vi "SignalAnalysisFrames.vi"() -> ()   [LabVIEW 2019]
uses:
  <vilib>/Analysis/4window.llb/windowTd.ctl
  <vilib>/Analysis/baseanly.llb/Mean (DBL).vi
  <vilib>/measure/maspectr.llb/FFT Spectrum (Mag-Phase) for N Chan.vi
  <vilib>/addons/Sound and Vibration/Order Analysis/Tach Process/OAT Analog Tacho Process (1 Tacho).vi
  <vilib>/addons/Sound and Vibration/Order Analysis/Resample Order Tracking/OAT Convert to Even Angle Signal (N Channels).vi
  <vilib>/addons/Sound and Vibration/Order Analysis/Utility/OAT Output Triggered Even Angle Signal (N Channels).vi
  <vilib>/addons/Sound and Vibration/Order Analysis/Resample Order Tracking/OAT Order Power Spectrum (N Channels).vi
  <vilib>/Analysis/NI_AALPro.lvlib
  <vilib>/measure/NI_MAPro.lvlib
  <vilib>/Analysis/NI_AALBase.lvlib
  <vilib>/addons/Sound and Vibration/Order Analysis/Tach Process/SoundVib_TachProcess.lvlib
  <vilib>/addons/Sound and Vibration/Order Analysis/Resample Order Tracking/SoundVib_OrderTracking.lvlib
  <vilib>/addons/Sound and Vibration/Order Analysis/Utility/SoundVib_OAUtility.lvlib
panel:
  out "Rotational speed [RPM] 2":dbl format="%0.2f"
  out "Rotational speed [RPM]":dbl format="%0.2f"
  in  "dł. ramki [s]":dbl=1.0
  in  "czułość 2 [V/g]":dbl=0.206
  in  "Skalować sygnał 2?":bool=TRUE
  in  "file path 2":path
  out "FFT analizator":cluster{"f0":dbl, "df":dbl, "magnitude":dbl[]}[](graph)
  out "order power spectrum 2":T1(graph)
  in  "FFT averaging":T2={"averaging mode"=enum."Vector averaging", "weighting mode"=enum."Exponential", "number of averages"=10}
  in  "Skalować sygnał 1?":bool
  out "order power spectrum":T1(graph)
  out "FFT karta pomiarowa":cluster{"f0":dbl, "df":dbl, "magnitude":dbl[]}[](graph)
  in  "order resolution":dbl=0.1 min=0.0 format="%.2f"
  in  "pulse/revolution (1)":i32=4
  in  "czułość 1 [V/g]":dbl=1.0
  in  "fs [Hz]":i64=5120
  in  "file path":path
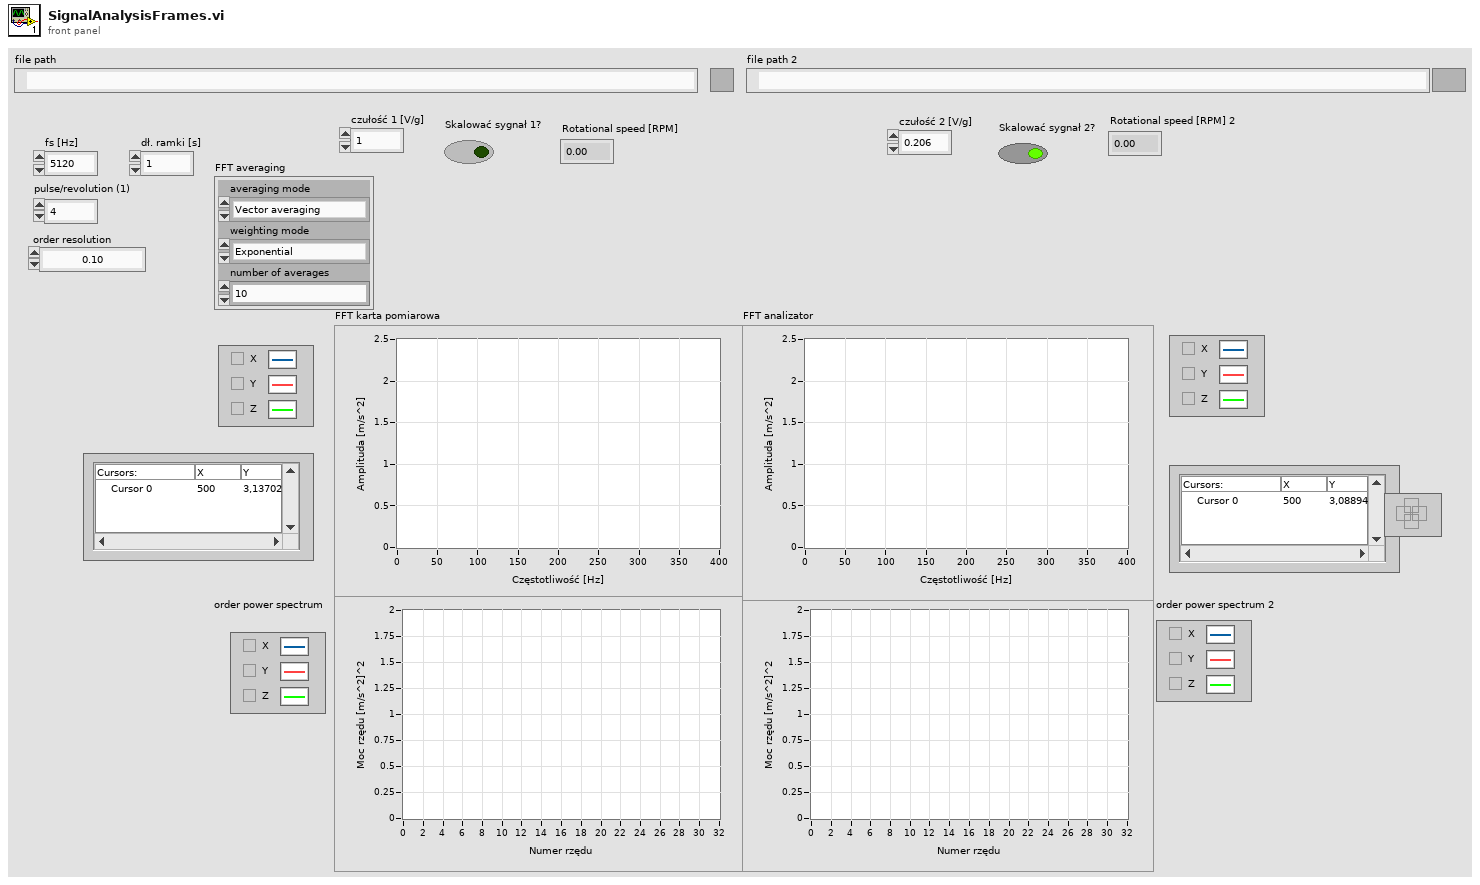
[diagram p1: front panel]
types:
  T1 = cluster{"order 0":dbl, "delta order":dbl, "magnitude":dbl[]}[]
  T2 = cluster{"averaging mode":enum16{"No averaging", "Vector averaging", "RMS averaging", "Peak hold"}, "weighting mode":enum16{"Linear", "Exponential"}, "number of averages":u32}
  T3 = enum16{"open", "open or create", "create or replace", "create", "open (read-only)"}
  T4 = enum16{"No averaging", "Vector averaging", "RMS averaging", "Peak hold"}
  T5 = cluster{"averaging mode":enum16{"No averaging", "Vector averaging", "RMS averaging", "Peak hold"}, "weighting mode":enum16{"Linear", "Exponential"}, "number of averages":u32, "linear mode":enum16{"One shot", "Auto restart"}}
  T6 = typedef "NI_AALPro.lvlib/windowTd.ctl" = u32
  T7 = typedef "SoundVib_TachProcess.lvlib/speed profile.ctl" = cluster{"time [s]":dbl[], "speed [RPM]":dbl[]}
  T8 = typedef "svc_Resampled Channel Info.ctl" = cluster{"channel name":string, "description":string, " channel info":T9}
  T9 = typedef "svc_Channel Info.ctl" = cluster{"sensor sensitivity":dbl, "engineering units":T10, "dB reference":dbl, "custom label":string, "weighting filter":T11, "pregain":dbl}
  T10 = typedef "svc_Engineering Units Text Ring.ctl" = u16
  T11 = typedef "svc_Weighting Filter Text Ring.ctl" = u16
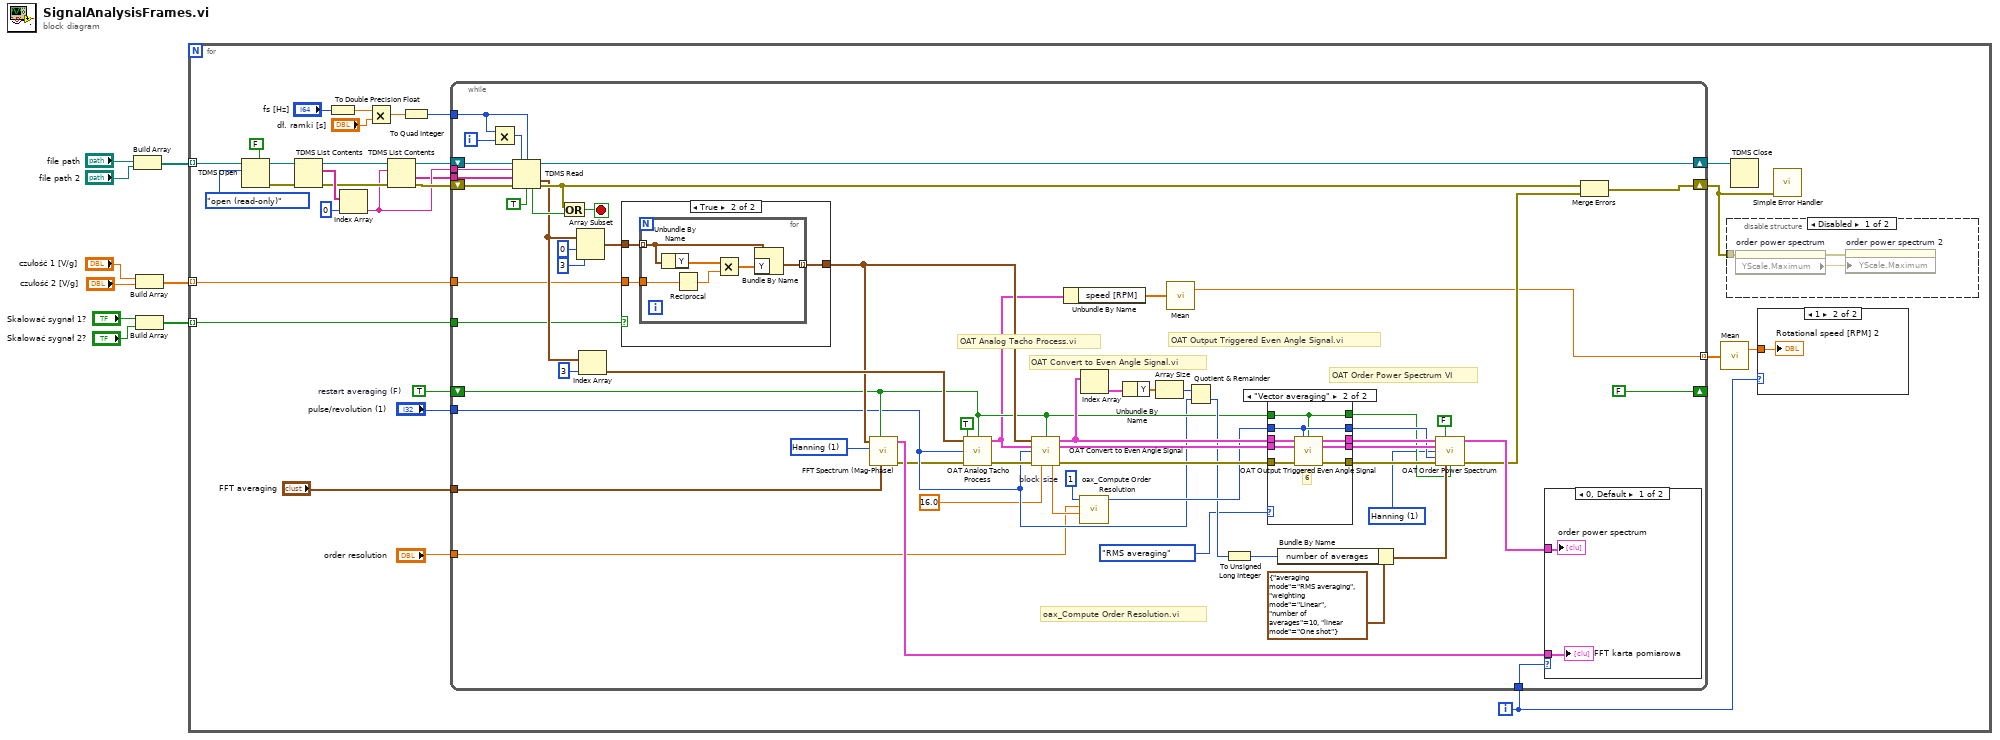
[diagram p0: block diagram]
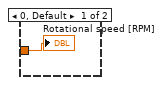
[diagram p3: hidden frame]
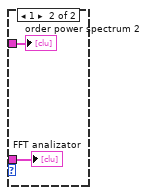
[diagram p5: hidden frame]
diagram:
  n1 = Build Array("file path", "file path 2") -> (w5:path[])
  n2 = Build Array("czułość 1 [V/g]", "czułość 2 [V/g]") -> (w3:dbl[])
  n3 = Build Array("Skalować sygnał 1?", "Skalować sygnał 2?") -> (w1:bool[])
  n4 = for {
    tunnel: w3 -> [w23] mode=indexing
    tunnel: w1 -> [w20] mode=indexing
    tunnel: w5 -> [w19] mode=indexing
    i -> [w12]
    w24 = TRUE  # restart averaging (F)
    n5 = TDMS Open(5:FALSE ("create index file? (T)"), 10:T3."open (read-only)" ("operation (0:open)"), 11:w19) -> (0:w28:errorcluster, 3:w29:refnum<k34>)  [unwired: 4 in]
    n6 = TDMS List Contents(4:w28, 7:w29) -> (0:w33:errorcluster, 2:w36:string[], 3:w35:refnum<k34>)  [unwired: 1 in, 1 out]
    n7 = To Double Precision Float(number="fs [Hz]") -> (double precision float=w15:dbl)
    n8 = Index Array(array=w36, index=0) -> (element=w31:string)
    n9 = Multiply(x=w15, y="dł. ramki [s]") -> (x*y=w18:dbl)
    n10 = TDMS List Contents(4:w33, 6:w31, 7:w35) -> (0:w32:errorcluster, 1:w30:string[], 3:w34:refnum<k34>)  [unwired: 1 out]
    n11 = To Quad Integer(1:w18) -> (0:w16:i64)
    n12 = while {
      tunnel: w31 -> [w101]
      tunnel: w30 -> [w100]
      shift-right: [w98] -> w27
      shift-left: w34 -> [w103]
      shift-right: [w83] -> w11
      shift-left: w32 -> [w102]
      tunnel: w16 -> [w92]
      shift-right: [FALSE ("restart averaging (F)")] -> _
      shift-left: w24 -> [w55]
      tunnel: w23 -> [w84]
      tunnel: "pulse/revolution (1)" -> [w54]
      tunnel: "order resolution" -> [w51]
      tunnel: w20 -> [w82]
      tunnel: "FFT averaging" -> [w81]
      tunnel: w12 -> [w79]
      tunnel: [w44] -> w14 mode=indexing
      i -> [w94]
      stop <- w97 stop-if-true
      w49 = u32 1 items=["None"=0, "Hanning"=1, "Hamming"=2, "Blackman-Harris"=3, "Exact Blackman"=4, "Blackman"=5, "Flat Top"=6, "4 Term B-Harris"=7, "7 Term B-Harris"=8, "Low Sidelobe"=9, "Gaussian"=62] ("window")
      w76 = 1  # block size
      w88 = T6 1 items=["Rectangle"=0, "Hanning"=1, "Hamming"=2, "Blackman-Harris"=3, "Exact Blackman"=4, "Blackman"=5, "Flat Top"=6, "4 Term B-Harris "=7, "7 Term B-Harris"=8, "Low Sidelobe"=9, "Blackman Nuttall"=11, "Triangle"=30, "Bartlett-Hanning"=31, "Bohman"=32, "Parzen"=33, "Welch"=34, "Kaiser"=60, "Dolph-Chebyshev"=61, "Gaussian"=62] ("window")
      # "oax_Compute Order Resolution.vi"
      # "OAT Order Power Spectrum VI"
      # "OAT Output Triggered Even Angle Signal.vi"
      # "OAT Convert to Even Angle Signal.vi"
      # "OAT Analog Tacho Process.vi"
      n13 = Multiply(x=w92, y=w94) -> (x*y=w93:i64)
      n14 = TDMS Read(0:w103, 1:w93, 2:w92, 5:w101, 7:w100, 11:w102, 13:TRUE ("return channels in file order? (F)")) -> (4:w98:refnum<k34>, 10:w86:waveform(dbl)[], 14:w95:bool, 15:w96:errorcluster)  [unwired: 1 in, 2 out]
      n15 = Or(x=w96, y=w95) -> (x .or. y?=w97:bool)
      n16 = Array Subset(array=w86, index=0, length=3) -> (w87:waveform(dbl)[])
      n17 = Index Array(array=w86, index=3) -> (element=w57:waveform(dbl))
      n18 = case shown="True" w82 {
        tunnel: w87 -> [w121 w124]
        tunnel: [w121 w123] -> w56
        tunnel: w84 -> [_ w122]
        frame False {
        }
        frame True {
          n19 = for {
            tunnel: w124 -> [w129] mode=indexing
            tunnel: [w128] -> w123 mode=indexing
            tunnel: w122 -> [w125]
            n20 = Unbundle By Name(w129) -> ("Y"=w130:dbl[])
            n21 = Reciprocal(x=w125) -> (1/x=w127:dbl)
            n22 = Multiply(x=w130, y=w127) -> (x*y=w126:dbl[])
            n23 = Bundle By Name(cluster=w129, "Y"=w126) -> (w128:waveform(dbl))
          }
        }
      }
      n24 = call-poly <vilib>:"FFT Spectrum (Mag-Phase).vi"("averaging parameters"=w81, "restart averaging (F)"=w55, "window"=w88, "time signals"=w56) -> ("error out"=w53:errorcluster, "magnitudes"=w80:cluster{"f0":dbl, "df":dbl, "magnitude":dbl[]}[])  [unwired: 3 in, 3 out]
      n25 = call-poly <vilib>:"OAT Analog Tacho Process.vi"("analog tacho signal"=w57, "missing pulses? (no:F)"=TRUE, "reset? (F)"=w55, "pulse/revolution (1)"=w54, "error in (no error)"=w53) -> ("speed profile"=w46:T7, "error out"=w74:errorcluster)  [unwired: 6 in, 3 out]
      n26 = call-poly <vilib>:"OAT Convert to Even Angle Signal.vi"("scaled signals [EU]"=w56, "reset? (F)"=w55, "speed profile"=w46, "pulse/revolution (1)"=w54, "error in (no error)"=w74, "max order (auto)"=16.0) -> ("even-angle signals"=w68:cluster{"r0":dbl, "dr":dbl, "Y":dbl[]}[], "even-angle channel info"=w72:T8[], "actual max order"=w75:dbl, "error out"=w73:errorcluster)  [unwired: 5 in, 1 out]
      n27 = Unbundle By Name(w46) -> ("speed [RPM]"=w45:dbl[])
      n28 = call <vilib>:"oax_Compute Order Resolution.vi"("actual max order"=w75, "order resolution"=w51, "block size"=w76) -> ("block size out"=w66:i32)  [unwired: 7 in, 1 out]
      n29 = Index Array(array=w68) -> (element=w71:cluster{"r0":dbl, "dr":dbl, "Y":dbl[]})  [unwired: 1 in]
      n30 = Unbundle By Name(w71) -> ("Y"=w70:dbl[])
      n31 = Array Size(array=w70) -> (size(s)=w69:i32)
      n32 = call-poly <vilib>:"Mean.vi"("X"=w45) -> ("mean"=w44:dbl)  [unwired: 1 out]
      n33 = Quotient & Remainder(x=w69, y=w54) -> (floor(x/y)=w61:i32)  [unwired: 1 out]
      n34 = To Unsigned Long Integer(number=w61) -> (unsigned 32bit integer=w60:u32)
      n35 = case shown="\"Vector averaging\"" T4."RMS averaging" ("averaging mode") {
        tunnel: w73 -> [w107 w116]
        tunnel: [w107 w115] -> w62
        tunnel: w66 -> [w108 w114]
        tunnel: [w108 w114] -> w63
        tunnel: w68 -> [w105 w113]
        tunnel: w72 -> [w106 w112]
        tunnel: [w106 w110] -> w64
        tunnel: [w105 w111] -> w65
        tunnel: w55 -> [w104 w109]
        tunnel: [w104 w109] -> w58
        frame "No averaging", Default {
        }
        frame "Vector averaging" {
          # "6"
          n36 = call-poly <vilib>:"OAT Output Triggered Even Angle Signal.vi"("even-angle signals"=w113, "block size"=w114, "reset? (F)"=w109, "even-angle channel info"=w112, "error in (no error)"=w116) -> ("triggered even-angle signals"=w111:cluster{"r0":dbl, "dr":dbl, "Y":dbl[]}[], "even-angle channel info out"=w110:T8[], "error out"=w115:errorcluster)  [unwired: 8 in]
        }
      }
      n37 = Bundle By Name(cluster=T5 {"averaging mode"=enum."RMS averaging", "weighting mode"=enum."Linear", "number of averages"=10, "linear mode"=enum."One shot"} ("averaging parameters"), "number of averages"=w60) -> (w59:T5)
      n38 = call-poly <vilib>:"OAT Order Power Spectrum.vi"("even-angle signals"=w65, "dB on? (T)"=FALSE, "even-angle channel info"=w64, "window"=w49, "block size"=w63, "error in (no error)"=w62, "averaging parameters"=w59, "restart averaging? (F)"=w58) -> ("order power spectra"=w48:T1, "error out"=w47:errorcluster)  [unwired: 1 in, 5 out]
      n39 = case shown="0, Default" w79 {
        tunnel: w48 -> [w118 w120]
        tunnel: w80 -> [w117 w119]
        frame 0, Default {
          "order power spectrum" <- w118
          "FFT karta pomiarowa" <- w117
        }
        frame 1 {
          "order power spectrum 2" <- w120
          "FFT analizator" <- w119
        }
      }
      n40 = Merge Errors(w96, w47) -> (w83:errorcluster)
    }
    n41 = call-poly <vilib>:"Mean.vi"("X"=w14) -> ("mean"=w13:dbl)  [unwired: 1 out]
    n42 = disable-structure shown="Disabled" {
      disable-tunnel: w11 -> [w40 _]
      frame Disabled {
        n43 = property on="order power spectrum" class="WFGraph (strict)"(error in=w40) -> (error out=w41:errorcluster, "YScale.Maximum"=w39:dbl)  [unwired: 1 in, 1 out]
        n44 = property on="order power spectrum 2" class="WFGraph (strict)"(error in=w41, "YScale.Maximum"=w39) -> ()  [unwired: 1 in, 2 out]
      }
      frame Enabled {
      }
    }
    n45 = TDMS Close(11:w27) -> ()  [unwired: 1 in, 2 out]
    n46 = case shown="1" w12 {
      tunnel: w13 -> [w42 w43]
      frame 0, Default {
        "Rotational speed [RPM]" <- w42
      }
      frame 1 {
        "Rotational speed [RPM] 2" <- w43
      }
    }
    n47 = call <vilib>:"Simple Error Handler.vi"("error in (no error)"=w11) -> ()  [unwired: 4 in, 5 out]
  }
